vi "Scratch.vi"() -> ()   [LabVIEW 2016]
uses:
  <vilib>/xnet/xnet.llb/XNET Write (Signal Single-point).vi
panel:
  out "error out":errorcluster
  in  "stop":bool
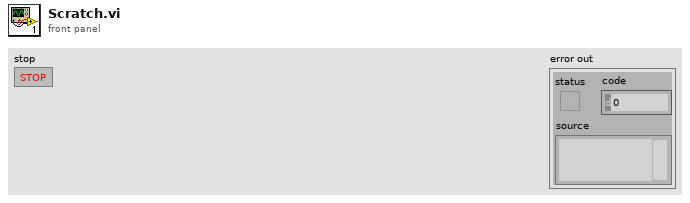
[diagram p1: front panel]
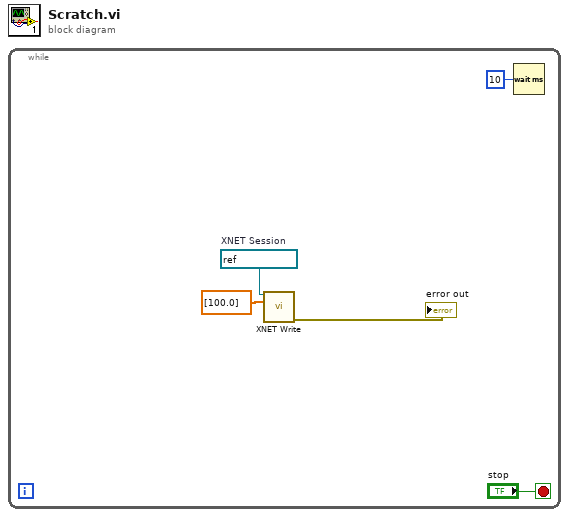
[diagram p0: block diagram]
diagram:
  n1 = while {
    stop <- "stop" stop-if-true
    w4 = refnum<k21> "Recv_test"  # XNET Session
    n2 = call-poly <vilib>:"XNET Write.vi"("session in"=w4, "data"=dbl[] [100.0]) -> ("error out"=→"error out":errorcluster)  [unwired: 12 in, 1 out]
    n3 = Wait (ms)(milliseconds to wait=u32 10) -> ()  [unwired: 1 out]
  }
